vi "main_serial_communication_3.vi"() -> ()   [LabVIEW 2015]
panel:
  out "호퍼2":sgl(graph)
  out "flow3":sgl
  out "Center":sgl(graph)
  out "flow2":sgl
  out "호퍼1":sgl(graph)
  out "flow":sgl
  in  "호퍼":enum16{"1", "2"}(ring)=enum."2"
  in  "delay (ms)":u32=500
  in  "?":bool
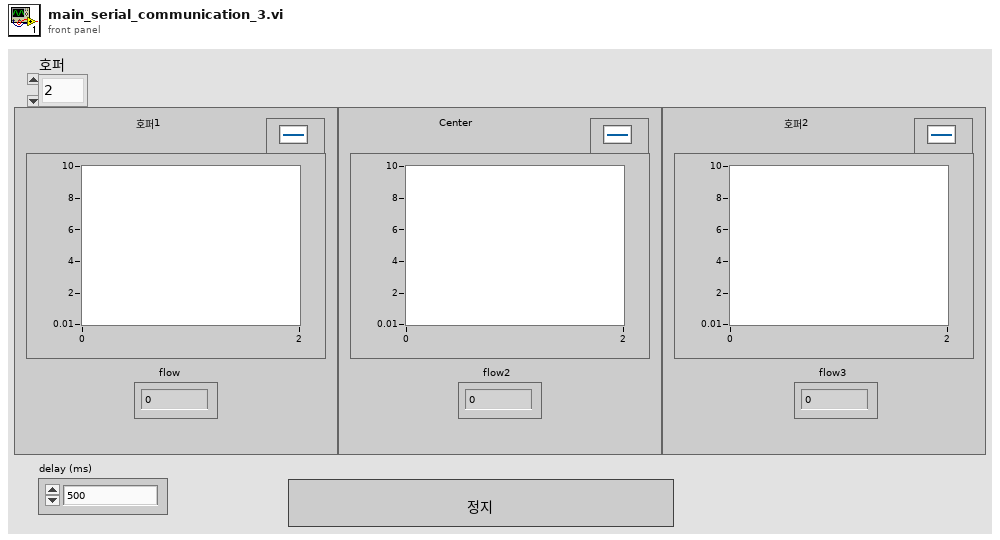
[diagram p1: front panel]
types:
  T1 = enum16{"open", "replace", "create", "open or create", "replace or create", "replace or create with confirmation"}
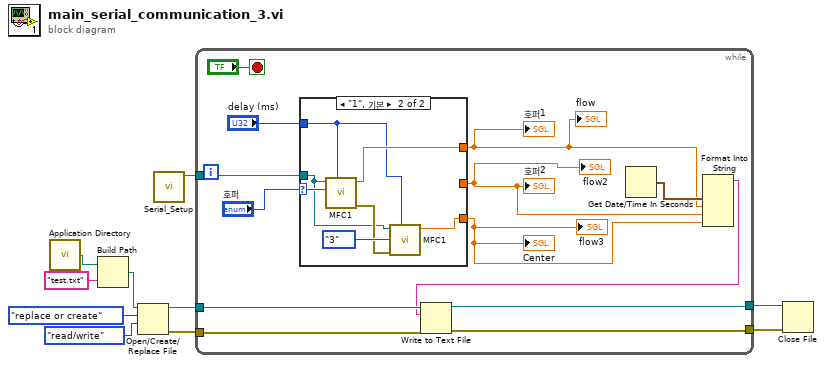
[diagram p0: block diagram]
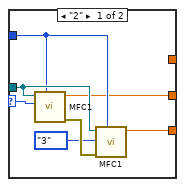
[diagram p2: hidden frame]
diagram:
  n1 = call <vilib>:"Application Directory.vi"() -> ("Application Directory"=w9:path)
  n2 = Build Path(base path=w9, name or relative path="test.txt" ("이름 또는 상대 경로")) -> (appended path=w7:path)
  n3 = Open/Create/Replace File(file path (use dialog)=w7, operation (0:open)=T1."replace or create" ("동작(0:open)"), access (0:read/write)=enum16{"read/write", "read-only", "write-only"}."read/write" ("접근(0:읽기/쓰기)")) -> (refnum out=w3:refnum<file>, error out=w4:errorcluster)  [unwired: 3 in, 1 out]
  n4 = call "Serial_Setup.vi"() -> ("VISA resource name out"=w10:refnum<visa-resource-name>)  [unwired: 10 in, 1 out]
  n5 = while {
    tunnel: w10 -> [w22]
    tunnel: w4 -> [w19]
    tunnel: w3 -> [w18]
    tunnel: [w17] -> w2
    tunnel: [w16] -> w1
    stop <- "?" stop-if-true
    n6 = case shown="\"1\", 기본" "호퍼" {
      selector: "호퍼" -> [w30 w36]
      tunnel: w22 -> [w28 w33]
      tunnel: [_ w37] -> w13
      tunnel: "delay (ms)" -> [w26 w32]
      tunnel: [w25 w31] -> w11
      tunnel: [w24 _] -> w12
      frame "2" {
        n7 = call "MFC1.vi"("delay (ms)"=w26, "열거형"=w30, "Port"=w28) -> ("error out"=w29:errorcluster, "flow"=w24:sgl)  [unwired: 7 in]
        n8 = call "MFC1.vi"("delay (ms)"=w26, "Error In"=w29, "열거형"=enum16{"1", "2", "3"}."3", "Port"=w28) -> ("flow"=w25:sgl)  [unwired: 6 in, 1 out]
      }
      frame "1", Default {
        n9 = call "MFC1.vi"("delay (ms)"=w32, "열거형"=w36, "Port"=w33) -> ("error out"=w34:errorcluster, "flow"=w37:sgl)  [unwired: 7 in]
        n10 = call "MFC1.vi"("delay (ms)"=w32, "Error In"=w34, "열거형"=enum16{"1", "2", "3"}."3", "Port"=w33) -> ("flow"=w31:sgl)  [unwired: 6 in, 1 out]
      }
    }
    "flow" <- w13
    "호퍼1" <- w13
    "flow2" <- w12
    "Center" <- w11
    "flow3" <- w11
    "호퍼2" <- w12
    n11 = Get Date/Time In Seconds() -> (seconds since 1Jan1904=w15:timestamp)
    n12 = Format Into String(w15, w13, w12, w11) -> (resulting string=w14:string)  [unwired: 3 in, 1 out]
    n13 = Write to Text File(file (use dialog)=w18, text=w14, error in=w19) -> (refnum out=w17:refnum<file>, error out=w16:errorcluster)  [unwired: 1 in, 1 out]
  }
  n14 = Close File(refnum=w2, error in=w1) -> ()  [unwired: 2 out]
